vi "UsingLoops.vi"() -> ()   [LabVIEW 2018]
panel:
  in  "milliseconds to wait":u32
  in  "stop":bool
  out "Thermometer (C)":dbl(slide) scale=0.0..100.0
  in  "Temperature (F)":dbl(slide) scale=0.0..200.0
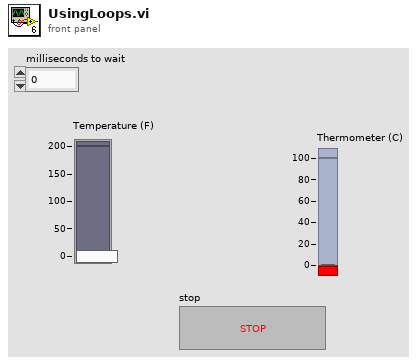
[diagram p1: front panel]
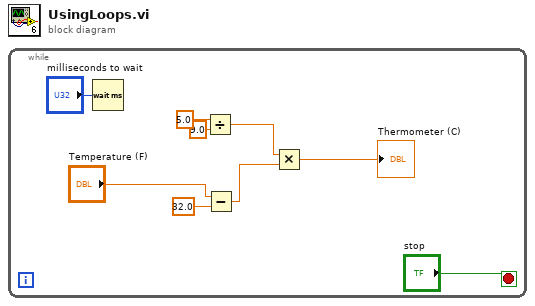
[diagram p0: block diagram]
diagram:
  n1 = while {
    stop <- "stop" stop-if-true
    n2 = Wait (ms)(milliseconds to wait="milliseconds to wait") -> ()  [unwired: 1 out]
    n3 = Divide(x=5.0, y=9.0) -> (x/y=w7:dbl)
    n4 = Subtract(x="Temperature (F)", y=32.0) -> (x-y=w6:dbl)
    n5 = Multiply(x=w7, y=w6) -> (x*y=→"Thermometer (C)":dbl)
  }
